vi "ARITHMETIC.vi"() -> ()   [LabVIEW 2018]
panel:
  out "DIV":dbl
  out "MUL":dbl
  out "SUB":dbl
  out "ADD":dbl
  in  "Numeric 2":dbl
  in  "Numeric":dbl
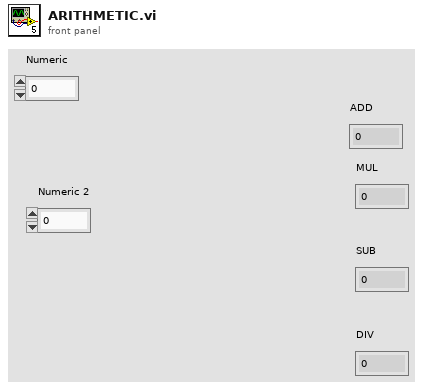
[diagram p1: front panel]
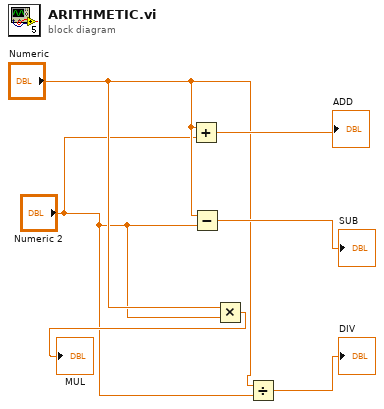
[diagram p0: block diagram]
diagram:
  n1 = Add(x="Numeric", y="Numeric 2") -> (x+y=→"ADD":dbl)
  n2 = Subtract(x="Numeric", y="Numeric 2") -> (x-y=→"SUB":dbl)
  n3 = Multiply(x="Numeric", y="Numeric 2") -> (x*y=→"MUL":dbl)
  n4 = Divide(x="Numeric", y="Numeric 2") -> (x/y=→"DIV":dbl)
